vi "m1m3ssdtView.vi"   [LabVIEW 2015, in "M1M3SSSTViews.lvlib"]
uses:
  M1M3SSSTViews.lvlib
  CommandFactory/CommandFactory.lvclass
  UserEvents/UserEvents.lvclass
  UserEvents/UserEvents.lvclass/UserEvents.ctl
  Typedefs/CommandSelector.ctl
  Typedefs/StateSelector.ctl
  stiffnessGraphView.vi
  stiffnessSummaryView.vi
  Typedefs/M1M3SSSTypedefs.lvlib
  Controller/Controller.lvclass
  ConfigurationThisComponent/ConfigurationThisComponent.lvclass
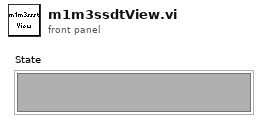
[diagram p1: front panel]
types:
  T1 = enum32{"invalid app kind", "Development System", "Run Time System", "Student Edition", "Embedded LabVIEW", "Evaluation", "Custom"}
  T2 = typedef "M1M3SSSTypedefs.lvlib/PubDataEvents.ctl" = cluster{"State":refnum<user-event>, "ErrorCode":refnum<user-event>, "OutputData":refnum<user-event>, "InputData":refnum<user-event>, "ControllerData":refnum<user-event>, "TestStatus":refnum<user-event>, "LogPath":refnum<user-event>, "StiffnessDataAssembly":refnum<user-event>, "PreconditioningCycle":refnum<user-event>}
  T3 = typedef "M1M3SSSTypedefs.lvlib/SubDataEvents.ctl" = cluster{"Command":refnum<user-event>}
  T4 = cluster{"Event Registration Refnum":refnum<event-registration>, "Event Registration Refnum":refnum<event-registration>}
  T5 = typedef "M1M3SSSTypedefs.lvlib/CommandSelector.ctl" = enum16{"ClearError", "Exit", "StandBy", "Start", "StartTest", "StopTest", "Update"}
  T6 = typedef "M1M3SSSTypedefs.lvlib/StateSelector.ctl" = enum16{"FaultState", "OffState", "RampingUpPressurePState", "RampingUpPressureSTState", "StandbyState", "StoppedState", "WaitingForSettledPState", "WaitingForSettledSTState"}
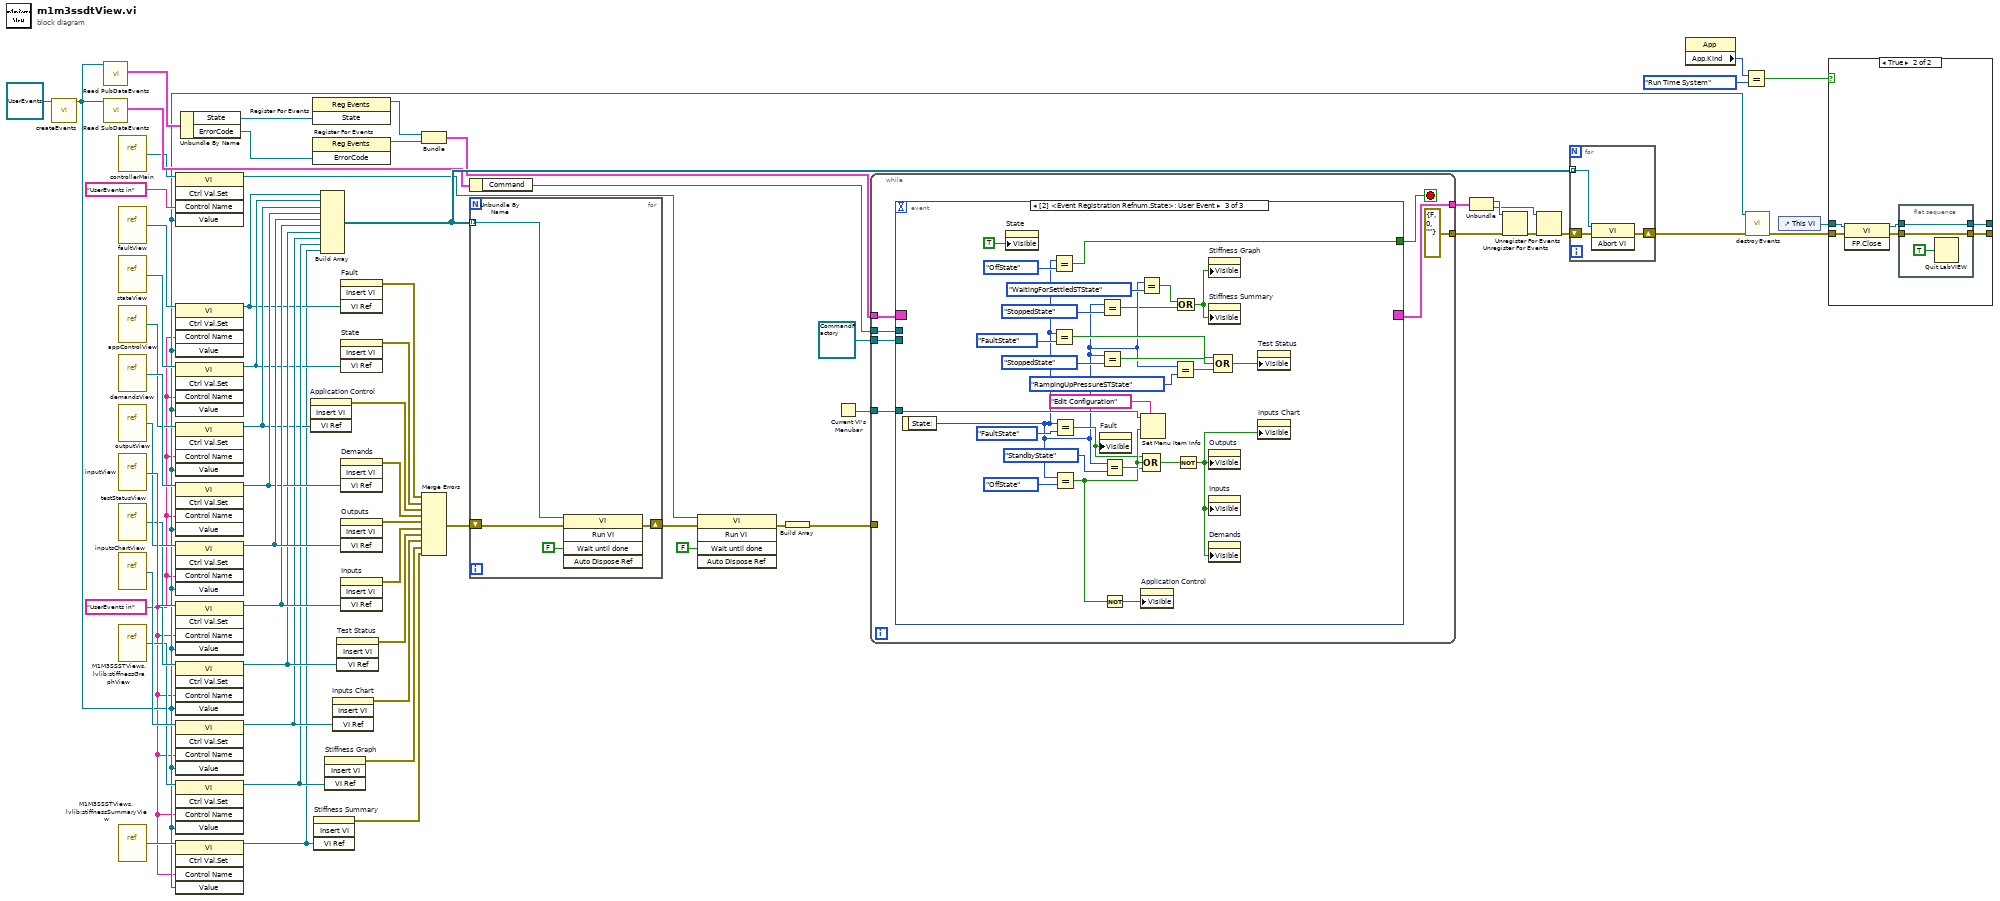
[diagram p0: block diagram]
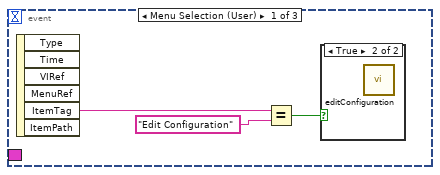
[diagram p3: hidden frame]
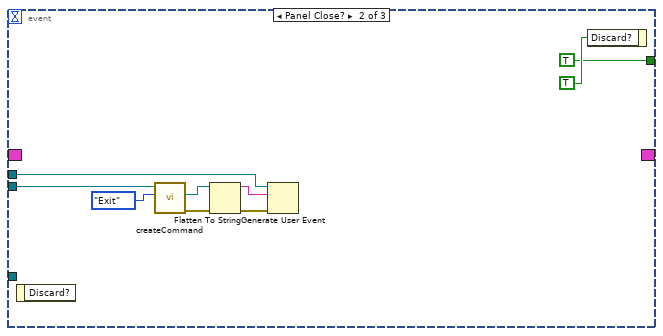
[diagram p5: hidden frame]
diagram:
  w3 = "UserEvents in" ("Control Name")
  n1 = call "createEvents.vi"("UserEvents in"=refnum<class "UserEvents.lvclass"> refnum) -> ("UserEvents out"=w4:refnum<class "UserEvents.lvclass">)  [unwired: 9 in, 1 out]
  n2 = call "Read PubDataEvents.vi"("UserEvents in"=w4) -> ("PubDataEvents"=w55:T2)  [unwired: 9 in, 1 out]
  n3 = call "Read SubDataEvents.vi"("UserEvents in"=w4) -> ("SubDataEvents"=w53:T3)  [unwired: 9 in, 1 out]
  n4 = vi-ref "controllerMain.vi"() -> (w46:refnum<vi>)
  n5 = vi-ref "faultView.vi"() -> (w12:refnum<vi>)
  n6 = vi-ref "stateView.vi"() -> (w15:refnum<vi>)
  n7 = vi-ref "appControlView.vi"() -> (w18:refnum<vi>)
  n8 = vi-ref "demandsView.vi"() -> (w30:refnum<vi>)
  n9 = vi-ref "outputView.vi"() -> (w35:refnum<vi>)
  n10 = vi-ref "inputView.vi"() -> (w43:refnum<vi>)
  n11 = vi-ref "testStatusView.vi"() -> (w27:refnum<vi>)
  n12 = vi-ref "inputsChartView.vi"() -> (w24:refnum<vi>)
  n13 = vi-ref "M1M3SSSTViews.lvlib:stiffnessGraphView.vi"() -> (w21:refnum<vi>)
  n14 = vi-ref "M1M3SSSTViews.lvlib:stiffnessSummaryView.vi"() -> (w5:refnum<vi>)
  n15 = invoke class="VI" method="Ctrl Val.Set"(reference=w46, "Control Name"="UserEvents in", "Value"=w4) -> (reference out=w44:refnum<vi>)  [unwired: 2 in, 4 out]
  n16 = invoke class="VI" method="Ctrl Val.Set"(reference=w12, "Control Name"=w3, "Value"=w4) -> (reference out=w11:refnum<vi>)  [unwired: 2 in, 4 out]
  n17 = invoke class="VI" method="Ctrl Val.Set"(reference=w15, "Control Name"=w3, "Value"=w4) -> (reference out=w14:refnum<vi>)  [unwired: 2 in, 4 out]
  n18 = invoke class="VI" method="Ctrl Val.Set"(reference=w18, "Control Name"=w3, "Value"=w4) -> (reference out=w16:refnum<vi>)  [unwired: 2 in, 4 out]
  n19 = invoke class="VI" method="Ctrl Val.Set"(reference=w30, "Control Name"=w3, "Value"=w4) -> (reference out=w29:refnum<vi>)  [unwired: 2 in, 4 out]
  n20 = invoke class="VI" method="Ctrl Val.Set"(reference=w35, "Control Name"=w3, "Value"=w4) -> (reference out=w34:refnum<vi>)  [unwired: 2 in, 4 out]
  n21 = invoke class="VI" method="Ctrl Val.Set"(reference=w43, "Control Name"=w3, "Value"=w4) -> (reference out=w33:refnum<vi>)  [unwired: 2 in, 4 out]
  n22 = invoke class="VI" method="Ctrl Val.Set"(reference=w27, "Control Name"=w3, "Value"=w4) -> (reference out=w26:refnum<vi>)  [unwired: 2 in, 4 out]
  n23 = invoke class="VI" method="Ctrl Val.Set"(reference=w24, "Control Name"=w3, "Value"=w4) -> (reference out=w22:refnum<vi>)  [unwired: 2 in, 4 out]
  n24 = invoke class="VI" method="Ctrl Val.Set"(reference=w21, "Control Name"=w3, "Value"=w4) -> (reference out=w20:refnum<vi>)  [unwired: 2 in, 4 out]
  n25 = invoke class="VI" method="Ctrl Val.Set"(reference=w5, "Control Name"=w3, "Value"=w4) -> (reference out=w1:refnum<vi>)  [unwired: 2 in, 4 out]
  n26 = Unbundle By Name(w55) -> ("State"=w51:refnum<user-event>, "ErrorCode"=w49:refnum<user-event>)
  n27 = invoke on="Application Control" class="SubPnl" method="Insert VI"("VI Ref"=w16) -> (error out=w17:errorcluster)  [unwired: 3 in, 3 out]
  n28 = register-events(w51) -> (reference out=w50:refnum<event-registration>)  [unwired: 2 in, 1 out]
  n29 = register-events(w49) -> (reference out=w48:refnum<event-registration>)  [unwired: 2 in, 1 out]
  n30 = invoke on="Stiffness Summary" class="SubPnl" method="Insert VI"("VI Ref"=w1) -> (error out=w2:errorcluster)  [unwired: 3 in, 3 out]
  n31 = Build Array(w11, w14, w16, w29, w34, w33, w26, w22, w20, w1) -> (w58:refnum<vi>[])
  n32 = invoke on="Stiffness Graph" class="SubPnl" method="Insert VI"("VI Ref"=w20) -> (error out=w19:errorcluster)  [unwired: 3 in, 3 out]
  n33 = invoke on="Inputs Chart" class="SubPnl" method="Insert VI"("VI Ref"=w22) -> (error out=w23:errorcluster)  [unwired: 3 in, 3 out]
  n34 = invoke on="Test Status" class="SubPnl" method="Insert VI"("VI Ref"=w26) -> (error out=w25:errorcluster)  [unwired: 3 in, 3 out]
  n35 = invoke on="Fault" class="SubPnl" method="Insert VI"("VI Ref"=w11) -> (error out=w10:errorcluster)  [unwired: 3 in, 3 out]
  n36 = invoke on="State" class="SubPnl" method="Insert VI"("VI Ref"=w14) -> (error out=w13:errorcluster)  [unwired: 3 in, 3 out]
  n37 = invoke on="Demands" class="SubPanel" method="Insert VI"("VI Ref"=w29) -> (error out=w28:errorcluster)  [unwired: 3 in, 3 out]
  n38 = invoke on="Outputs" class="SubPanel" method="Insert VI"("VI Ref"=w34) -> (error out=w61:errorcluster)  [unwired: 3 in, 3 out]
  n39 = invoke on="Inputs" class="SubPnl" method="Insert VI"("VI Ref"=w33) -> (error out=w60:errorcluster)  [unwired: 3 in, 3 out]
  n40 = Bundle("Event Registration Refnum"=w50, "Event Registration Refnum"=w48) -> (w41:T4)  [unwired: 1 in]
  n41 = Merge Errors(w10, w13, w17, w28, w61, w60, w25, w23, w19, w2) -> (w59:errorcluster)
  n42 = Unbundle By Name(w53) -> ("Command"=w52:refnum<user-event>)
  n43 = for {
    tunnel: w58 -> [w68] mode=indexing
    shift-right: [w67] -> w6
    shift-left: w59 -> [w66]
    n44 = invoke class="VI" method="Run VI"(reference=w68, error in=w66, "Wait until done"=FALSE ("Wait Until Done")) -> (error out=w67:errorcluster)  [unwired: 2 in, 4 out]
  }
  n45 = invoke class="VI" method="Run VI"(reference=w44, error in=w6, "Wait until done"=FALSE ("Wait Until Done")) -> (error out=w31:errorcluster)  [unwired: 2 in, 4 out]
  n46 = Build Array(w31) -> (w7:errorcluster[])
  n47 = Current VI's Menubar() -> (w56:refnum<k9>)
  n48 = while {
    tunnel: refnum<class "CommandFactory.lvclass"> refnum ("CommandFactory.lvclass") -> [w72]
    tunnel: [errorcluster {"status"=FALSE, "code"=0, "source"=""} ("error out")] -> w42
    tunnel: w56 -> [w70]
    tunnel: w41 -> [w74]
    tunnel: w52 -> [w71]
    tunnel: [w69] -> w40
    tunnel: w7 -> [_]
    stop <- w73 stop-if-true
    n49 = event shown="[2] <Event Registration Refnum.State>: User Event" {
      selector: w74 -> [_ _ _]
      dyn-events: [_ _ _] -> w69
      timeout: _ -> [_ _ _]
      tunnel: [_ TRUE w108] -> w73
      tunnel: w72 -> [_ w82 _]
      tunnel: w71 -> [_ w79 _]
      tunnel: w70 -> [_ _ w110]
      event Menu Selection (User) {
        n50 = event-data() -> ("ItemTag"=w76:string)  [unwired: 1 in, 5 out]
        n51 = Equal?(x=w76, y="Edit Configuration") -> (x = y?=w78:bool)
        n52 = case shown="True" w78 {
          frame False {
          }
          frame True {
            n53 = call "editConfiguration.vi"() -> ()  [unwired: 10 in, 2 out]
          }
        }
      }
      event Panel Close? {
        n54 = event-data() -> ()  [unwired: 1 in, 1 out]
        n55 = call-dynamic "createCommand.vi"("Command"=CommandSelector."Exit", "CommandFactory in"=w82) -> ("error out"=w87:errorcluster, "command"=w86:refnum<class "Command.lvclass">)  [unwired: 7 in, 1 out]
        n56 = Flatten To String(anything=w86, error in (no error)=w87) -> (data string=w80:string, error out=w81:errorcluster)  [unwired: 2 in, 1 out]
        n57 = Generate User Event(user event=w79, event data cluster=w80, error in=w81) -> ()  [unwired: 1 in, 2 out]
        n58 = event-data("Discard?"=TRUE) -> ()  [unwired: 1 in, 1 out]
      }
      event User Event {
        n59 = event-data() -> ("State:"=w91:T6)  [unwired: 1 in]
        n60 = property on="State" class="SubPnl"("Visible"=TRUE) -> ()  [unwired: 2 in, 2 out]
        n61 = Equal?(x=w91, y=StateSelector."OffState") -> (x = y?=w108:bool)
        n62 = Equal?(x=w91, y=StateSelector."FaultState") -> (x = y?=w102:bool)
        n63 = Equal?(x=w91, y=StateSelector."FaultState") -> (x = y?=w95:bool)
        n64 = Equal?(x=w91, y=StateSelector."OffState") -> (x = y?=w97:bool)
        n65 = property on="Fault" class="SubPnl"("Visible"=w95) -> ()  [unwired: 2 in, 2 out]
        n66 = Equal?(x=w91, y=StateSelector."StoppedState") -> (x = y?=w89:bool)
        n67 = Equal?(x=w91, y=StateSelector."StoppedState") -> (x = y?=w101:bool)
        n68 = Equal?(x=w91, y=StateSelector."StandbyState") -> (x = y?=w107:bool)
        n69 = Not(x=w97) -> (.not. x?=w98:bool)
        n70 = Equal?(x=w91, y=StateSelector."WaitingForSettledSTState") -> (x = y?=w90:bool)
        n71 = Set Menu Item Info(7:"Edit Configuration" ("item name"), 9:w107, 11:w110) -> ()  [unwired: 4 in, 2 out]
        n72 = property on="Application Control" class="SubPnl"("Visible"=w98) -> ()  [unwired: 2 in, 2 out]
        n73 = Compound Arithmetic op=OR(w95, w107, w97) -> (w106:bool)
        n74 = Equal?(x=w91, y=StateSelector."RampingUpPressureSTState") -> (x = y?=w100:bool)
        n75 = Or(x=w90, y=w89) -> (x .or. y?=w88:bool)
        n76 = Not(x=w106) -> (.not. x?=w94:bool)
        n77 = property on="Stiffness Graph" class="SubPnl"("Visible"=w88) -> ()  [unwired: 2 in, 2 out]
        n78 = property on="Stiffness Summary" class="SubPnl"("Visible"=w88) -> ()  [unwired: 2 in, 2 out]
        n79 = property on="Outputs" class="SubPnl"("Visible"=w94) -> ()  [unwired: 2 in, 2 out]
        n80 = property on="Inputs" class="SubPnl"("Visible"=w94) -> ()  [unwired: 2 in, 2 out]
        n81 = property on="Demands" class="SubPnl"("Visible"=w94) -> ()  [unwired: 2 in, 2 out]
        n82 = Compound Arithmetic op=OR(w102, w101, w100) -> (w99:bool)
        n83 = property on="Test Status" class="SubPnl"("Visible"=w99) -> ()  [unwired: 2 in, 2 out]
        n84 = property on="Inputs Chart" class="SubPnl"("Visible"=w94) -> ()  [unwired: 2 in, 2 out]
      }
    }
  }
  n85 = Unbundle(w40) -> ("Event Registration Refnum"=w39:refnum<event-registration>, "Event Registration Refnum"=w37:refnum<event-registration>)
  n86 = Unregister For Events(event registration refnum=w39, error in=w42) -> (error out=w38:errorcluster)
  n87 = Unregister For Events(event registration refnum=w37, error in=w38) -> (error out=w36:errorcluster)
  n88 = for {
    tunnel: w58 -> [w117] mode=indexing
    shift-right: [w115] -> w32
    shift-left: w36 -> [w116]
    n89 = invoke class="VI" method="Abort VI"(reference=w117, error in=w116) -> (error out=w115:errorcluster)  [unwired: 1 in, 2 out]
  }
  n90 = property class="App"() -> ("App.Kind"=w64:T1)  [unwired: 2 in, 2 out]
  n91 = Equal?(x=w64, y=T1."Run Time System") -> (x = y?=w62:bool)
  n92 = call "destroyEvents.vi"("error in (no error)"=w32, "UserEvents in"=w4) -> ("error out"=w8:errorcluster)  [unwired: 8 in, 1 out]
  n93 = control-ref of="This VI"() -> (w9:refnum<vi>)
  n94 = case shown="True" w62 {
    tunnel: w9 -> [w119 w125]
    tunnel: w8 -> [w118 w124]
    tunnel: [w119 w122] -> _
    tunnel: [w118 w120] -> _
    frame False {
    }
    frame True {
      n95 = invoke class="VI" method="FP.Close"(reference=w125, error in=w124) -> (reference out=w121:refnum<vi>, error out=w123:errorcluster)  [unwired: 1 in, 1 out]
      n96 = flat-sequence {
        tunnel: w123 -> [w126]
        tunnel: [w127] -> w122
        tunnel: w121 -> [w127]
        tunnel: [w126] -> w120
        frame #0 {
          n97 = Quit LabVIEW(quit? (T)=TRUE) -> ()
        }
      }
    }
  }
